vi "Configuration - INI Path-Default--Const.vi"() -> (3 "Default INI Path":string)   [LabVIEW 2017, in "Communications Library.lvlib"]
uses:
  Communications Library.lvlib
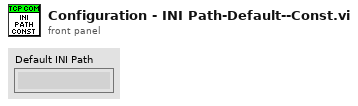
[diagram p1: front panel]
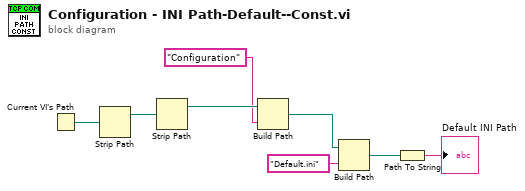
[diagram p0: block diagram]
diagram:
  n1 = Current VI's Path() -> (path=w8:path)
  n2 = Strip Path(path=w8) -> (stripped path=w7:path)  [unwired: 1 out]
  n3 = Strip Path(path=w7) -> (stripped path=w6:path)  [unwired: 1 out]
  n4 = Build Path(base path=w6, name or relative path="Configuration") -> (appended path=w3:path)
  n5 = Build Path(base path=w3, name or relative path="Default.ini") -> (appended path=w2:path)
  n6 = Path To String(path=w2) -> (string=→"Default INI Path":string)
